vi "Test Actor.vi"() -> ()   [LabVIEW 2014, in "Generic Power Analyzer.lvlib" / "Tektronix PA1000.lvlib" / "Tektronix PA1000.lvclass"]
uses:
  Tektronix PA1000.lvclass
  <vilib>/ActorFramework/Message Queue/Message Queue.lvclass/Message Queue.ctl
  <vilib>/ActorFramework/Message Enqueuer/Message Priority.ctl
  <vilib>/ActorFramework/Message Enqueuer/Message Enqueuer.lvclass/Message Enqueuer.ctl
  <vilib>/ActorFramework/Message Enqueuer/Enqueue.vi
  <vilib>/ActorFramework/Message Priority Queue/Priority Enqueue.vi
  Generic Instrument Messages/Send Stop Event Msg/Send Stop Event Msg.lvclass
  <vilib>/ActorFramework/Message Queue/Message Queue.lvclass
  <vilib>/ActorFramework/Actor/Actor.lvclass
  <vilib>/ActorFramework/Message Enqueuer/Message Enqueuer.lvclass
panel:
  out "error out":errorcluster
  in  "Stop Button":bool
  in  "VISA resource name":refnum<visa-resource-name>
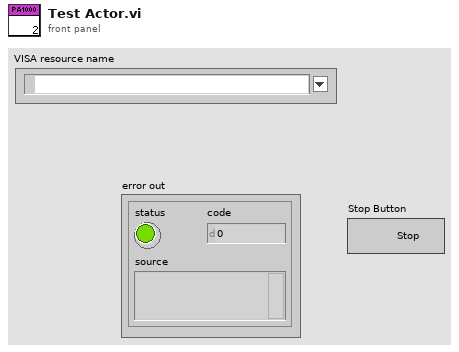
[diagram p1: front panel]
types:
  T1 = typedef "Actor Framework.lvlib/Message Enqueuer.lvclass/Message Priority.ctl" = enum16{"Low", "Normal", "High"}
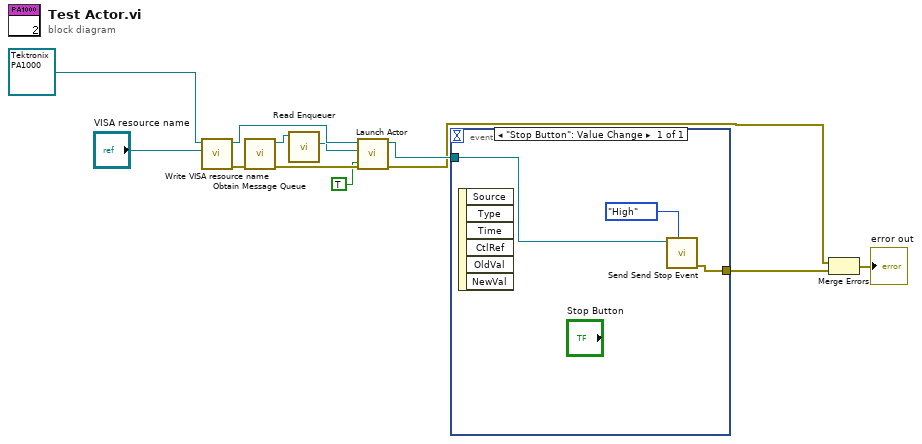
[diagram p0: block diagram]
diagram:
  n1 = call-dynamic "Write VISA resource name.vi"("VISA resource name"="VISA resource name", "Generic Instrument in"=refnum<class "Tektronix PA1000.lvclass"> refnum ("Generic Power Analyzer.lvlib:Tektronix PA1000.lvlib:Tektronix PA1000.lvclass")) -> ("error out"=w11:errorcluster, "Generic Instrument out"=w10:refnum<class "Tektronix PA1000.lvclass">)  [unwired: 8 in]
  n2 = call <vilib>:"Obtain Message Queue.vi"("error in (no error)"=w11) -> ("error out"=w12:errorcluster, "Message Queue"=w7:refnum<class "Message Queue.lvclass">)  [unwired: 9 in]
  n3 = call <vilib>:"Read Enqueuer.vi"("Message Queue"=w7) -> ("Message Enqueuer"=w8:refnum<class "Message Enqueuer.lvclass">)  [unwired: 10 in]
  n4 = call <vilib>:"Launch Actor.vi"("Open Actor Core front panel? (F)"=TRUE, "error in (no error)"=w12, "Actor-to-Caller Enqueuer"=w8, "Actor"=w10) -> ("error out"=w1:errorcluster, "Caller-To-Actor Enqueuer"=w4:refnum<class "Message Enqueuer.lvclass">)  [unwired: 6 in]
  n5 = event shown="[0] \"Stop Button\": Value Change" {
    selector: _ -> [_]
    dyn-events: _ -> [_]
    timeout: _ -> [_]
    tunnel: w4 -> [w15]
    tunnel: [w13] -> w2
    event "Stop Button": Value Change {
      n6 = event-data() -> ()  [unwired: 1 in, 6 out]
      n7 = call "Send Send Stop Event.vi"("Message Priority (Normal)"=Message_Priority."High", "Message Enqueuer"=w15) -> ("error out"=w13:errorcluster)  [unwired: 8 in, 1 out]
    }
  }
  n8 = Merge Errors(w1, w2) -> (→"error out":errorcluster)
